vi "MinSec2Sec.vi"(11 "duration (mm:ss)":string) -> (2 "duration DBL":dbl, 3 "duration (s)":string)   [LabVIEW 2015]
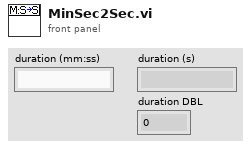
[diagram p1: front panel]
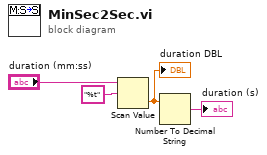
[diagram p0: block diagram]
diagram:
  n1 = Scan Value(string="duration (mm:ss)", format string="%t") -> (value=w2:dbl)  [unwired: 1 in, 1 out]
  "duration DBL" <- w2
  n2 = Number To Decimal String(number=w2) -> (decimal integer string=→"duration (s)":string)  [unwired: 1 in]
